vi "PH_AWG-510.set modified data.vi"(0 "i ref in":refnum<vi>, 2 "i attribute":T1={"GUI Refs"={"Delete"=refnum, "Trigger Settings"=refnum, "Start Device"=refnum, "Instrument Information"=refnum, "Lock Frontpanel"=refnum, "Waveform Pattern File"=refnum, "Initialize"=refnum, "Output Settings"=refnum}, "Instrument Information"={"VISA resource name"="", "Instrument Firmware Revision"="", "Manufacturer"="", "Model"="", "Serial Number"="", "Error Message"="0,\"No error\"\r\n", "Device Status"=enum."stopped"}, "Initialized?"=FALSE, "Current Settings"={"Trigger"={"Mode"=enum."Continuous", "Level (V)"=0.0, "External Source"=FALSE}, "Output Settings"={"Activate Channel"=FALSE, "VPP (V)"=0.0, "Clock (Hz)"=0.0, "File Name (Device)"="", "#1"=0, "#2"=0, "#3"=0, "#4"=0, "#5"=0, "#6"=0, "#7"=0, "#8"=0, "#9"=0, "#10"=0, "#11"=0, "#12"=0, "#13"=0, "#14"=0, "#15"=0, "#16"=0, "#17"=0, "#18"=0, "#19"=0, "#20"=0, "Offset (V)"=-1.0}}, "Wanted Settings"={"Trigger"={"Mode"=enum."Continuous", "Level (V)"=0.0, "External Source"=FALSE}, "Output Settings"={"Activate Channel"=FALSE, "VPP (V)"=0.0, "Clock (Hz)"=0.0, "File Name (Device)"="", "#1"=0, "#2"=0, "#3"=0, "#4"=0, "#5"=0, "#6"=0, "#7"=0, "#8"=0, "#9"=0, "#10"=0, "#11"=0, "#12"=0, "#13"=0, "#14"=0, "#15"=0, "#16"=0, "#17"=0, "#18"=0, "#19"=0, "#20"=0, "Offset (V)"=-1.0}}, "Device frontpanel locked?"=FALSE, "Default File Path"=path "D:/PCS/AWG"} {"Wanted Settings"."Output Settings"."#20" max=1023 step=1 scale=0.0..1023.0; "Wanted Settings"."Output Settings"."#19" max=1023 step=1 scale=0.0..1023.0; "Wanted Settings"."Output Settings"."#18" max=1023 step=1 scale=0.0..1023.0; "Wanted Settings"."Output Settings"."#17" max=1023 step=1 scale=0.0..1023.0; "Wanted Settings"."Output Settings"."#16" max=1023 step=1 scale=0.0..1023.0; "Wanted Settings"."Output Settings"."#15" max=1023 step=1 scale=0.0..1023.0; "Wanted Settings"."Output Settings"."#14" max=1023 step=1 scale=0.0..1023.0; "Wanted Settings"."Output Settings"."#13" max=1023 step=1 scale=0.0..1023.0; "Wanted Settings"."Output Settings"."#12" max=1023 step=1 scale=0.0..1023.0; "Wanted Settings"."Output Settings"."#11" max=1023 step=1 scale=0.0..1023.0; "Wanted Settings"."Output Settings"."#10" max=1023 step=1 scale=0.0..1023.0; "Wanted Settings"."Output Settings"."#9" max=1023 step=1 scale=0.0..1023.0; "Wanted Settings"."Output Settings"."#8" max=1023 step=1 scale=0.0..1023.0; "Wanted Settings"."Output Settings"."#7" max=1023 step=1 scale=0.0..1023.0; "Wanted Settings"."Output Settings"."#6" max=1023 step=1 scale=0.0..1023.0; "Wanted Settings"."Output Settings"."#5" max=1023 step=1 scale=0.0..1023.0; "Wanted Settings"."Output Settings"."#4" max=1023 step=1 scale=0.0..1023.0; "Wanted Settings"."Output Settings"."#3" max=1023 step=1 scale=0.0..1023.0; "Wanted Settings"."Output Settings"."#2" max=1023 step=1 scale=0.0..1023.0; "Wanted Settings"."Output Settings"."#1" max=1023 step=1 scale=0.0..1023.0; "Current Settings"."Output Settings"."#20" max=1023 step=1 scale=0.0..1023.0; "Current Settings"."Output Settings"."#19" max=1023 step=1 scale=0.0..1023.0; "Current Settings"."Output Settings"."#18" max=1023 step=1 scale=0.0..1023.0; "Current Settings"."Output Settings"."#17" max=1023 step=1 scale=0.0..1023.0; "Current Settings"."Output Settings"."#16" max=1023 step=1 scale=0.0..1023.0; "Current Settings"."Output Settings"."#15" max=1023 step=1 scale=0.0..1023.0; "Current Settings"."Output Settings"."#14" max=1023 step=1 scale=0.0..1023.0; "Current Settings"."Output Settings"."#13" max=1023 step=1 scale=0.0..1023.0; "Current Settings"."Output Settings"."#12" max=1023 step=1 scale=0.0..1023.0; "Current Settings"."Output Settings"."#11" max=1023 step=1 scale=0.0..1023.0; "Current Settings"."Output Settings"."#10" max=1023 step=1 scale=0.0..1023.0; "Current Settings"."Output Settings"."#9" max=1023 step=1 scale=0.0..1023.0; "Current Settings"."Output Settings"."#8" max=1023 step=1 scale=0.0..1023.0; "Current Settings"."Output Settings"."#7" max=1023 step=1 scale=0.0..1023.0; "Current Settings"."Output Settings"."#6" max=1023 step=1 scale=0.0..1023.0; "Current Settings"."Output Settings"."#5" max=1023 step=1 scale=0.0..1023.0; "Current Settings"."Output Settings"."#4" max=1023 step=1 scale=0.0..1023.0; "Current Settings"."Output Settings"."#3" max=1023 step=1 scale=0.0..1023.0; "Current Settings"."Output Settings"."#2" max=1023 step=1 scale=0.0..1023.0; "Current Settings"."Output Settings"."#1" max=1023 step=1 scale=0.0..1023.0}, 5 "error in (no error)":errorcluster) -> (14 "i ref out":refnum<vi>, 19 "error out":errorcluster)   [LabVIEW 2014, in "PH_AWG-510.lvlib"]
doc: "Writes the data into the attribute of an object. Then, the attribute dara are unlocked using the \"release\" method. Prior to calling THIS method, the attribute data must have been locked using the methods \"lock\" or \"get data to modify\".\n\n\nLicense Agreement for this software:\n\nCopyright (C)\nGesellschaft für Schwerionenforschung, GSI\nPlanckstr. 1\n64291 Darmstadt\nGermany\n\nContact: D.Beck@gsi.de \n\nThis program is free software; you can redistribute it and/or modify it under the terms of the GNU General Public License as published by the Free Software Foundation; either version 2 of the license, or (at your option) any later version.\n\nThis program is distributed in the hope that it will be useful, but WITHOUT ANY WARRANTY; without even the implied warranty of MERCHANTABILITY or FITNESS FOR A PARTICULAR PURPOSE. See the GNU General License for more details (http://www.gnu.org).\n\nGesellschaft für Schwerionenforschung, GSI\nPlanckstr. 1, 64291 Darmstadt, Germany\nFor all questions and ideas contact: M.Richter@gsi.de, H.Brand@gsi.de or D.Beck@gsi.de.\nLast update: 17-JUN-2004"
uses:
  PH_AWG-510.lvlib
  PH_AWG-510.i attribute.ctl
  PH_AWG-510.Trigger Settings.ctl
  PH_AWG-510.Instrument Information Dataset.ctl
  PH_AWG-510.Output Settings.ctl
  CSCore/CSObj/CSObj.lvlib
panel:
  # "Waveform Pattern"
  # "Waveform Pattern"
  # "Waveform Pattern"
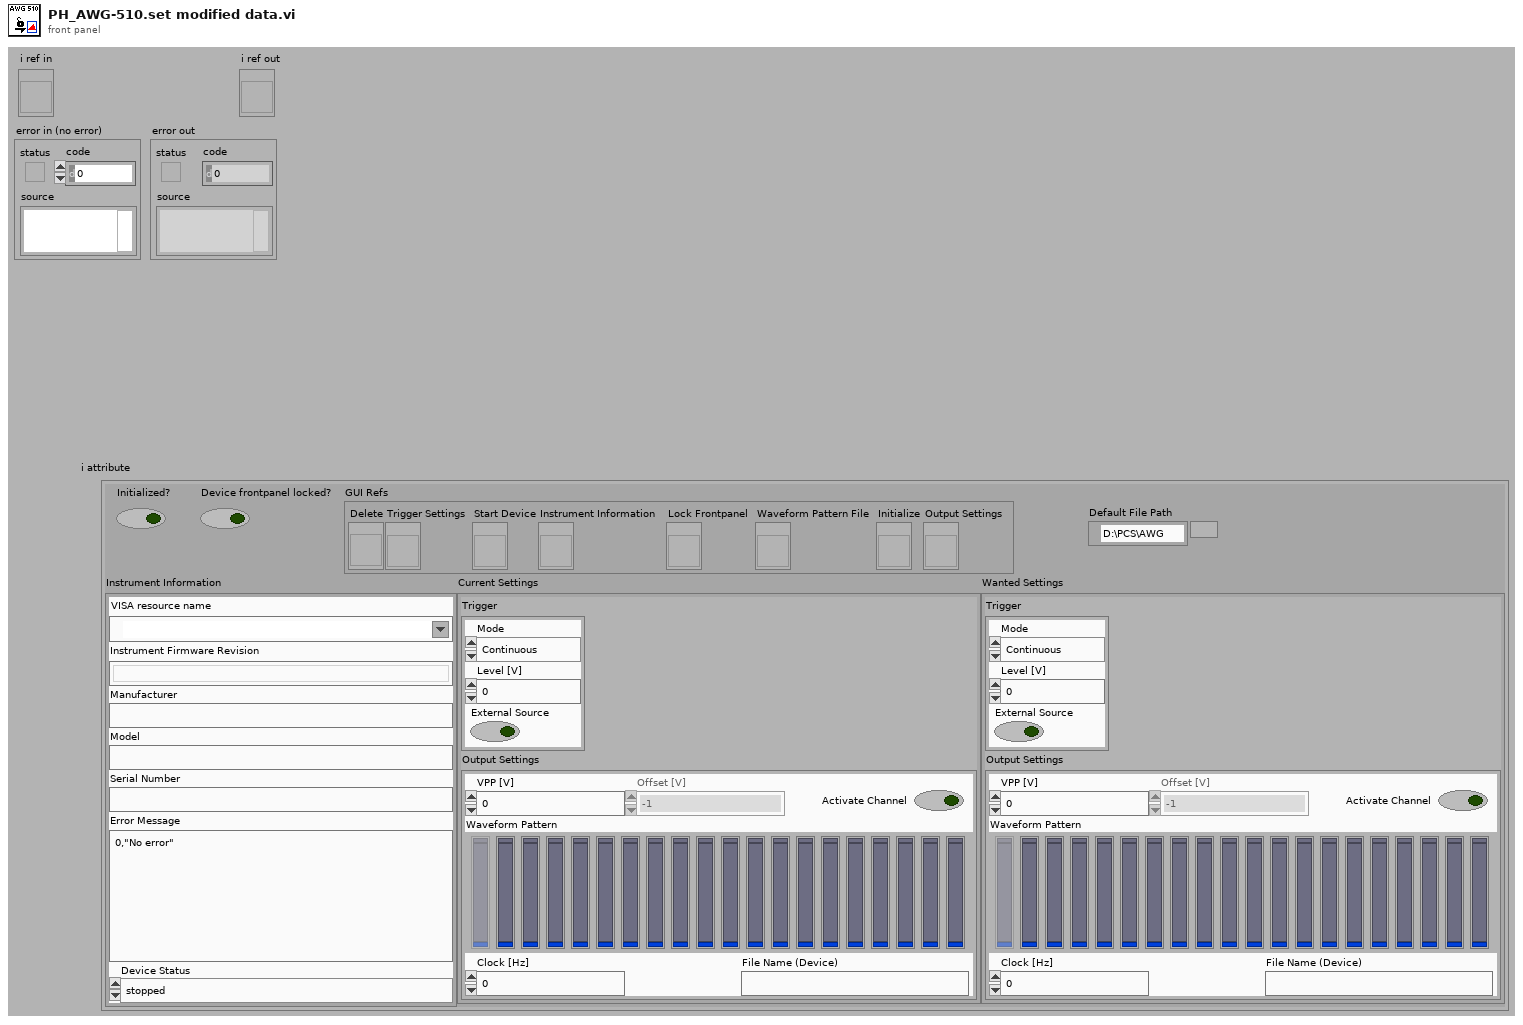
[diagram p1: front panel]
types:
  T1 = typedef "PH_AWG-510.lvlib/PH_AWG-510.i attribute.ctl" = cluster{"GUI Refs":cluster{"Delete":refnum<vi>, "Trigger Settings":refnum<vi>, "Start Device":refnum<vi>, "Instrument Information":refnum<vi>, "Lock Frontpanel":refnum<vi>, "Waveform Pattern File":refnum<vi>, "Initialize":refnum<vi>, "Output Settings":refnum<vi>}, "Instrument Information":T2, "Initialized?":bool, "Current Settings":cluster{"Trigger":T3, "Output Settings":T4}, "Wanted Settings":cluster{"Trigger":T3, "Output Settings":T4}, "Device frontpanel locked?":bool, "Default File Path":path}
  T2 = typedef "PH_AWG-510.lvlib/PH_AWG-510.Instrument Information Dataset.ctl" = cluster{"VISA resource name":refnum<visa-resource-name>, "Instrument Firmware Revision":string, "Manufacturer":string, "Model":string, "Serial Number":string, "Error Message":string, "Device Status":enum16{"stopped", "wating for trigger", "running", "Failure"}}
  T3 = typedef "PH_AWG-510.lvlib/PH_AWG-510.Trigger Settings.ctl" = cluster{"Mode":enum16{"Continuous", "Triggered", "Gated", "Enhanced"}, "Level (V)":dbl, "External Source":bool}
  T4 = typedef "PH_AWG-510.lvlib/PH_AWG-510.Output Settings.ctl" = cluster{"Activate Channel":bool, "VPP (V)":dbl, "Clock (Hz)":dbl, "File Name (Device)":string, "#1":u16, "#2":u16, "#3":u16, "#4":u16, "#5":u16, "#6":u16, "#7":u16, "#8":u16, "#9":u16, "#10":u16, "#11":u16, "#12":u16, "#13":u16, "#14":u16, "#15":u16, "#16":u16, "#17":u16, "#18":u16, "#19":u16, "#20":u16, "Offset (V)":dbl}
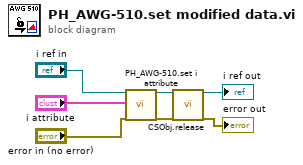
[diagram p0: block diagram]
diagram:
  n1 = call "PH_AWG-510.set i attribute.vi"("i ref in"="i ref in", "i attribute"="i attribute", "error in (no error)"="error in (no error)") -> ("i ref out"=w4:refnum<vi>, "error out"=w3:errorcluster)  [unwired: 15 in]
  n2 = call "CSObj.release.vi"("i ref in"=w4, "error in (no error)"=w3) -> ("i ref out"=→"i ref out":refnum<vi>, "error out"=→"error out":errorcluster)  [unwired: 16 in]
